vi "nth Derivative of Polynomial.vi"   [LabVIEW 2012, in "NI_AALPro.lvlib"]
doc: "Calculates the nth order derivative of <B>P(x)</B>. Wire data to the <B>P(x)</B> input to determine the polymorphic instance to use or manually select the instance."
uses:
  NI_AALPro.lvlib
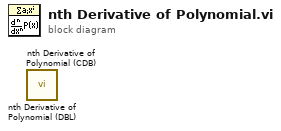
[diagram p0: block diagram]
diagram:
  n1 = call "nth Derivative of Polynomial (DBL).vi"() -> ()  [unwired: 10 in, 2 out]
  n2 = call "nth Derivative of Polynomial (CDB).vi"() -> ()  [unwired: 10 in, 2 out]
